vi "challenges.vi"(11 "project-param out 3":T1) -> (3 "project-param out 2":T1)   [LabVIEW 2019]
uses:
  Project Parameters.ctl
  <vilib>/numeric/Random Number (Range) I64.vi
  <vilib>/numeric/sub_Random U32.vi
panel:
  out "Utvalgt":string
  out "Selectables":string[](array[string])
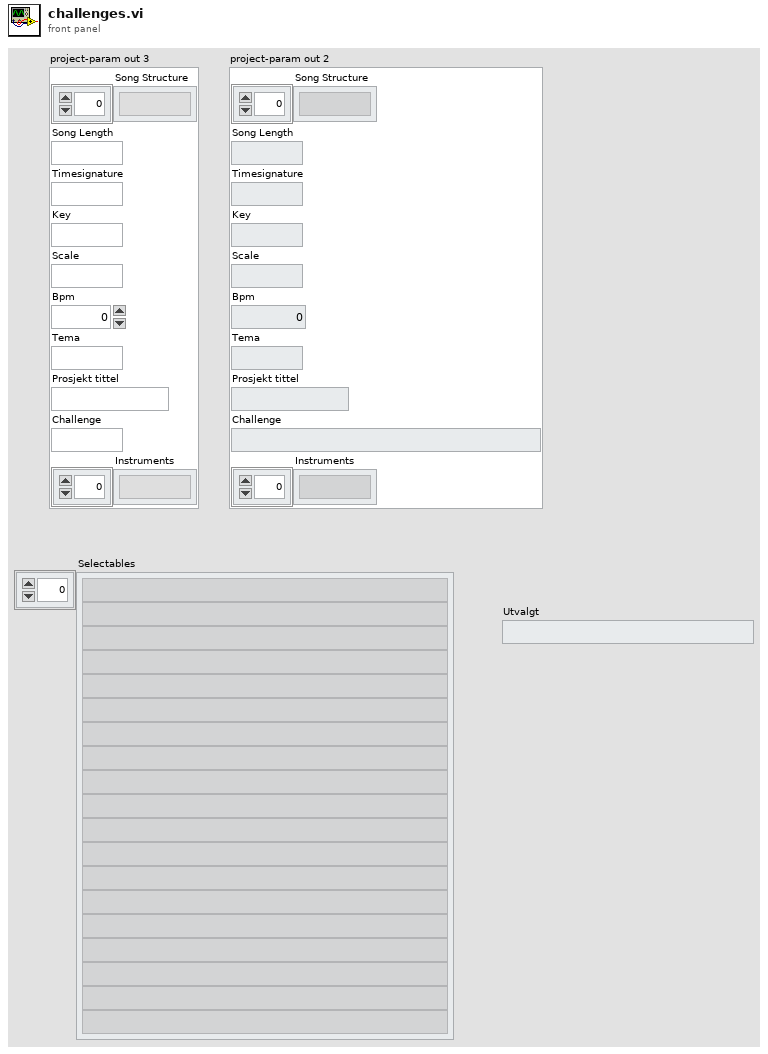
[diagram p1: front panel]
types:
  T1 = typedef "Project Parameters.ctl" = cluster{"Song Structure":string[], "Song Length":string, "Timesignature":string, "Key":string, "Scale":string, "Bpm":i32, "Tema":string, "Prosjekt tittel":string, "Challenge":string, "Instruments":string[]}
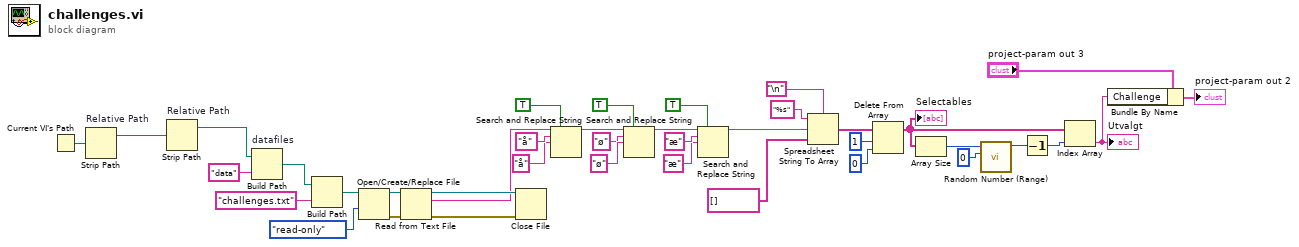
[diagram p0: block diagram]
diagram:
  n1 = Current VI's Path() -> (path=w38:path)
  n2 = Strip Path "Relative Path"(path=w38) -> (stripped path=w3:path)  [unwired: 1 out]
  n3 = Strip Path "Relative Path"(path=w3) -> (stripped path=w2:path)  [unwired: 1 out]
  n4 = Build Path "datafiles"(base path=w2, name or relative path="data") -> (appended path=w30:path)
  n5 = Build Path(base path=w30, name or relative path="challenges.txt") -> (appended path=w28:path)
  n6 = Open/Create/Replace File(file path (use dialog)=w28, access (0:read/write)=enum16{"read/write", "read-only", "write-only"}."read-only") -> (refnum out=w35:refnum<file>, error out=w34:errorcluster)  [unwired: 4 in, 1 out]
  n7 = Read from Text File(file (use dialog)=w35, error in=w34) -> (refnum out=w33:refnum<file>, text=w24:string, error out=w32:errorcluster)  [unwired: 2 in, 1 out]
  n8 = Close File(refnum=w33, error in=w32) -> ()  [unwired: 2 out]
  n9 = Search and Replace String(replace all?=TRUE ("replace all? (F)"), input string=w24, search string="å", replace string="å" ("replace string (\"\")")) -> (result string=w17:string)  [unwired: 4 in, 3 out]
  n10 = Search and Replace String(replace all?=TRUE ("replace all? (F)"), input string=w17, search string="ø", replace string="ø" ("replace string (\"\")")) -> (result string=w13:string)  [unwired: 4 in, 3 out]
  n11 = Search and Replace String(replace all?=TRUE ("replace all? (F)"), input string=w13, search string="æ", replace string="æ" ("replace string (\"\")")) -> (result string=w12:string)  [unwired: 4 in, 3 out]
  n12 = Spreadsheet String To Array(delimiter (Tab)="\n", format string="%s", spreadsheet string=w12, array type (2D Dbl)=string[] []) -> (array=w11:string[])
  n13 = Delete From Array(array=w11, length=1, index=0) -> (array with subset deleted=w6:string[])  [unwired: 1 out]
  "Selectables" <- w6
  n14 = Array Size(array=w6) -> (size(s)=w8:i32)
  n15 = call-poly <vilib>:"Random Number (Range).vi"("lower bound (-100)"=i64 0, "upper bound (100)"=w8) -> ("number"=w5:i64)  [unwired: 9 in]
  n16 = Decrement(x=w5) -> (x-1=w1:i64)
  n17 = Index Array(array=w6, index=w1) -> (element=w4:string)
  "Utvalgt" <- w4
  n18 = Bundle By Name(cluster="project-param out 3", "Challenge"=w4) -> (→"project-param out 2":T1)
